vi "write.vi"(8 "error in (no error)":errorcluster, 10 "writeString":string, 11 "SerialSimulator in":refnum<class "SerialSimulator.lvclass">) -> (0 "error out":errorcluster, 3 "SerialSimulator out":refnum<class "SerialSimulator.lvclass">)   [LabVIEW 2012, in "SerialSimulator.lvclass"]
uses:
  SerialSimulator.lvclass
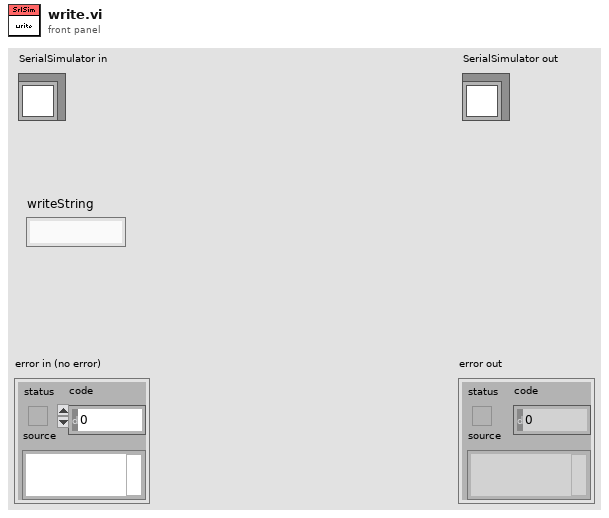
[diagram p1: front panel]
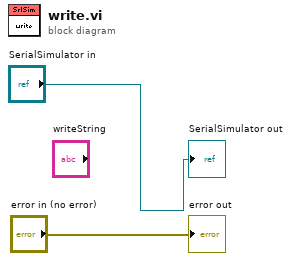
[diagram p0: block diagram]
diagram:
  "error out" <- "error in (no error)"
  "SerialSimulator out" <- "SerialSimulator in"
